vi "Get Path Data Size.vi"(10 "Data String":u8[](array[numeric])) -> (2 "Data Size":i32)   [LabVIEW 2017, in "Composition.lvlib"]
doc: "Gets the data size of a path"
uses:
  Composition.lvlib
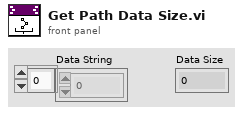
[diagram p1: front panel]
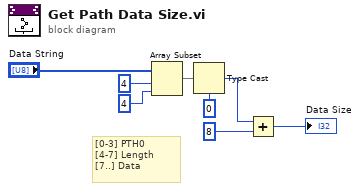
[diagram p0: block diagram]
diagram:
  # "[0-3] PTH0\n[4-7] Length\n[7..] Data"
  n1 = Array Subset(array="Data String", index=4, length=4) -> (w6:u8[])
  n2 = Type Cast(type=0, x=w6) -> (*(type *) &x=w7:i32)
  n3 = Add(x=w7, y=8) -> (x+y=→"Data Size":i32)
